vi "LDA_Power_spectrum.vi"(0 "U":dbl[](array[numeric]) format="%.2f", 1 "XTime":dbl[](array[numeric]) format="%.2f", 2 "Sampling frequency":sgl format="%.2f", 3 "Spectrum input array":dbl[](array[numeric]) format="%.2f", 4 "Block No":i32=1) -> (6 "Spectrum output array":dbl[](array[numeric]) format="%.2f")   [LabVIEW 2010]
panel:
  out "Average":T1(graph)
  out "Output Array":dbl format="%.2f"
  out "Spectra size":i32
  out "XY Graph":T1(graph)
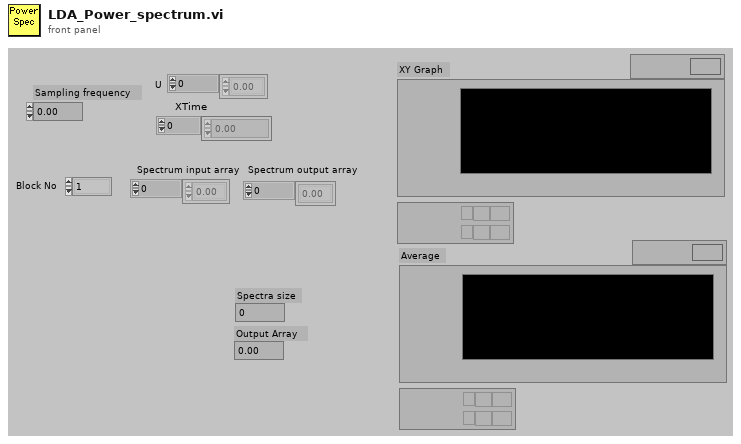
[diagram p1: front panel]
types:
  T1 = cluster{"Power Spectrum FFT {X}Frequency":dbl[], "Power Spectrum FFT {X}":dbl[]}
  T2 = cluster{"Power Spectrum FFT {X}Frequency":dbl[], dbl[]}
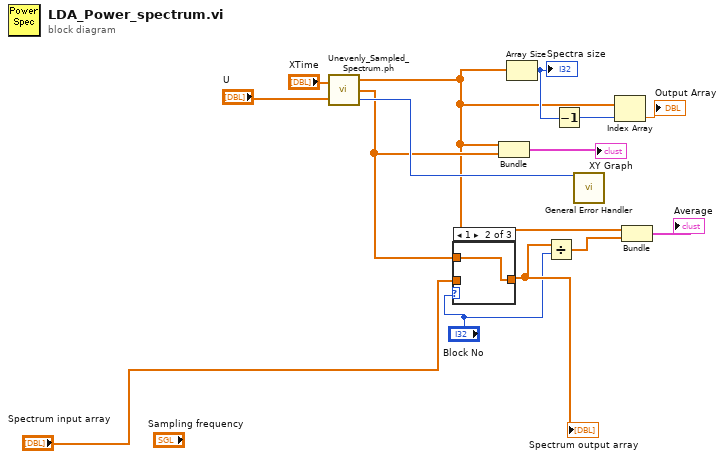
[diagram p0: block diagram]
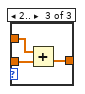
[diagram p3: hidden frame]
diagram:
  n1 = call "Unevenly_Sampled_Spectrum.ph.vi"("XTime"="XTime", "X"="U") -> ("Power Spectrum FFT {X}Frequency"=w3:dbl[], "Power Spectrum FFT {X}"=w6:dbl[], "error"=w11:i32)
  n2 = case shown="1" "Block No" {
    tunnel: [w15 w16 w19] -> w5
    tunnel: w6 -> [w15 w16 w18]
    tunnel: "Spectrum input array" -> [_ _ w17]
    frame ..0 {
    }
    frame 1 {
    }
    frame 2.. {
      n3 = Add(x=w18, y=w17) -> (x+y=w19:dbl[])
    }
  }
  "Spectrum output array" <- w5
  n4 = Bundle("Power Spectrum FFT {X}Frequency"=w3, "Power Spectrum FFT {X}"=w6) -> (→"XY Graph":T1)  [unwired: 1 in]
  n5 = Array Size(array=w3) -> (size(s)=w10:i32)
  "Spectra size" <- w10
  n6 = Divide(x=w5, y="Block No") -> (x/y=w2:dbl[])
  n7 = Decrement(x=w10) -> (x-1=w9:i32)
  n8 = call <vilib>:"General Error Handler.vi"("[error code] (0)"=w11) -> ()  [unwired: 10 in, 5 out]
  n9 = Index Array(array=w3, index=w9) -> (element=→"Output Array":dbl)
  n10 = Bundle("Power Spectrum FFT {X}Frequency"=w3, w2) -> (→"Average":T2)  [unwired: 1 in]
